vi "XIPIN_ILA_(ChipScope_Pro_-_Integrated_Logic_Analyzer)_1_05_a.vi"   [LabVIEW 2017]
doc: "The ChipScope Pro Series Integrated Logic Analyzer.\n------------------------------------\n<b>Need License</b> : No"
uses:
  <vilib>/rvi/XilinxIP/XIPIN_XNode/niFpgaXIPIN.xnode
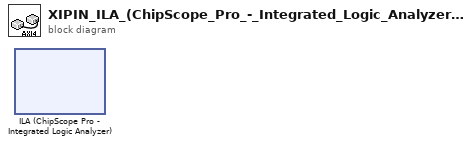
[diagram p0: block diagram]
diagram:
  n1 = xnode ("ILA (ChipScope Pro - Integrated Logic Analyzer)")() -> ()
